vi "Calibration Process.vi"() -> ()   [LabVIEW 2016]
uses:
  <vilib>/vision/Calibration.llb/Correction Learn Setup.ctl
  <vilib>/vision/Calibration.llb/Distortion Model Types.ctl
  <vilib>/vision/Calibration.llb/Error Statistics.ctl
  <vilib>/vision/Calibration.llb/Distortion Model.ctl
  <vilib>/vision/NI_Vision_Development_Module.lvlib
panel:
  out "Error Statistics":T1 {"% Distortion" format="%#_2g"; "Standard Deviation" format="%#_2g"; "Mean Error" format="%#_2g"; "Maximum Error" format="%#_2g"}
  out "Error Map":sgl[][](array[numeric]) format="%.4f"
  out "Calibration Axis Info":T2={"Origin Pixel"={"X"=0.0, "Y"=0.0}, "Angle Relative to Horizontal (deg)"=0.0, "X Axis Pixel"={"X"=0.0, "Y"=0.0}, "Axis Reference"=1} {"X Axis Pixel"."Y" format="%.2f"; "X Axis Pixel"."X" format="%.2f"; "Axis Reference" items=["Direct", "Indirect"]; "Angle Relative to Horizontal (deg)" format="%.2f"; "Origin Pixel"."Y" format="%.2f"; "Origin Pixel"."X" format="%.2f"}
  out "Calibration Learn Setup":T3={"Method"=4, "Distortion"=-1, "Corrected Image Scaling"=0, "Corrected Image Learn ROI"=0, "Learn Correction Table?"=FALSE} {"Distortion" items=["None"=-1, "Polynomial"=0, "Division"=1]; "Corrected Image Learn ROI" items=["Full Image ", "Calibration ROI", "ROI", "Calibration AND ROI", "Calibration OR ROI"]; "Corrected Image Scaling" items=["Scale to Preserve Area", "Scale to Fit"]; "Method" items=["Perspective", "Microplane", "Simple", "Corrected", "None"]}
  out "Src":T5(plugin-control)
  out "Bin":T5(plugin-control)
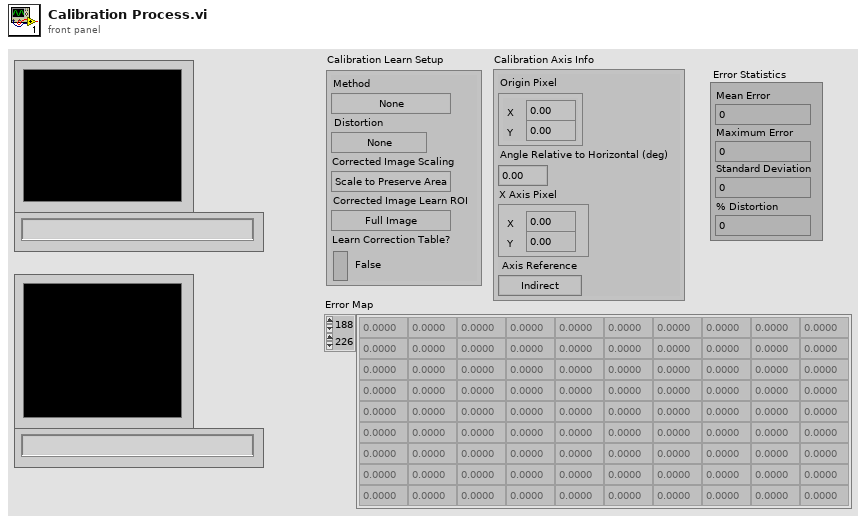
[diagram p1: front panel]
types:
  T1 = typedef "Error Statistics.ctl" = cluster{"Mean Error":dbl, "Maximum Error":dbl, "Standard Deviation":dbl, "% Distortion":dbl}
  T2 = cluster{"Origin Pixel":cluster{"X":sgl, "Y":sgl}, "Angle Relative to Horizontal (deg)":sgl, "X Axis Pixel":cluster{"X":sgl, "Y":sgl}, "Axis Reference":u32}
  T3 = typedef "Correction Learn Setup.ctl" = cluster{"Method":u32, "Distortion":T4, "Corrected Image Scaling":u32, "Corrected Image Learn ROI":u32, "Learn Correction Table?":bool}
  T4 = typedef "Distortion Model Types.ctl" = i32
  T5 = typedef "IMAQ Image.ctl" = refnum<image>
  T6 = typedef "Distortion Model.ctl" = cluster{"Distortion Model":T4, "Polynomial Model Setup":cluster{"Radial Coefficient":u32, "Tangential Coefficients ":bool}}
  T7 = typedef "Image Unit" = enum32{"Undefined", "Angström", "Micrometer", "Millimeter", "Centimeter", "Meter", "Kilometer", "Microinch", "Inch", "Feet", "Nautical miles", "Standard miles", "Steps"}
  T8 = typedef "Calibration Reference Points.ctl" = cluster{"Pixel Coordinates":cluster{"X":dbl, "Y":dbl}[], "Real World Coordinates":cluster{"X":dbl, "Y":dbl}[], "Unit":T7, "Image Size":cluster{"X":u32, "Y":u32}}
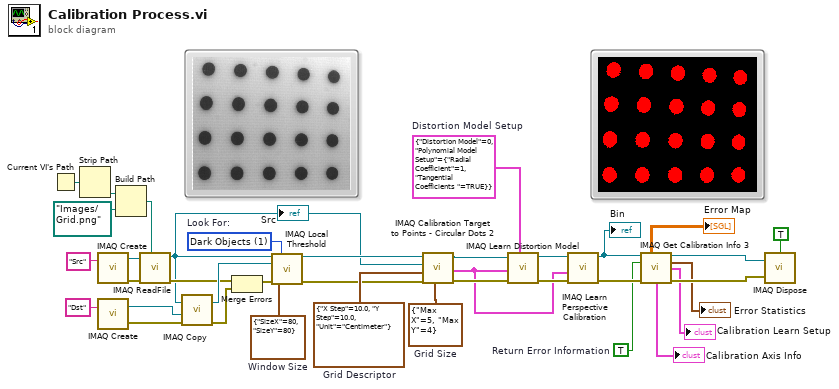
[diagram p0: block diagram]
diagram:
  w7 = TRUE  # Return Error Information
  w25 = T6 {"Distortion Model"=0, "Polynomial Model Setup"={"Radial Coefficient"=1, "Tangential Coefficients "=TRUE}}  # Distortion Model Setup
  w26 = cluster{"SizeX":i32, "SizeY":i32} {"SizeX"=80, "SizeY"=80}  # Window Size
  w27 = u32 1 items=["Bright Objects", "Dark Objects"]  # Look For:
  w28 = cluster{"Max X":u32, "Max Y":u32} {"Max X"=5, "Max Y"=4}  # Grid Size
  w30 = cluster{"X Step":sgl, "Y Step":sgl, "Unit":T7} {"X Step"=10.0, "Y Step"=10.0, "Unit"=enum."Centimeter"}  # Grid Descriptor
  n1 = Current VI's Path() -> (path=w33:path)
  n2 = Strip Path(path=w33) -> (stripped path=w32:path)  [unwired: 1 out]
  n3 = call "IMAQ Create"("Image Name"="Src") -> ("New Image"=w37:T5, "error out"=w36:errorcluster)  [unwired: 4 in]
  n4 = call "IMAQ Create"("Image Name"="Dst") -> ("New Image"=w15:T5, "error out"=w16:errorcluster)  [unwired: 4 in]
  n5 = Build Path(base path=w32, name or relative path=path "Images/Grid.png" ("prompt")) -> (appended path=w31:path)
  n6 = call "IMAQ ReadFile"("File Path"=w31, "error in (no error)"=w36, "Image"=w37) -> ("error out"=w12:errorcluster, "Image Out"=w6:T5)  [unwired: 4 in, 3 out]
  "Src" <- w6
  n7 = call "IMAQ Copy"("error in (no error)"=w16, "Image Dst"=w15, "Image Src"=w6) -> ("error out"=w11:errorcluster, "Image Dst Out"=w14:T5)  [unwired: 3 in]
  n8 = Merge Errors(w12, w11) -> (w10:errorcluster)
  n9 = call "IMAQ Local Threshold"("Image Src"=w6, "Look For (Bright Objects)"=w27, "Image Dst"=w14, "Window Size (32x32)"=w26, "error in (no error)"=w10) -> ("Image Dst Out"=w13:T5, "error out"=w22:errorcluster)  [unwired: 9 in]
  n10 = call "IMAQ Calibration Target to Points - Circular Dots 2"("Grid Size"=w28, "error in (no error)"=w22, "Grid Descriptor"=w30, "Grayscale Image"=w6, "Target Image"=w13) -> ("error out"=w21:errorcluster, "Reference Points"=w20:T8, "Target Image (dup)"=w5:T5)  [unwired: 4 in]
  n11 = call "IMAQ Learn Distortion Model"("Distortion Model Setup"=w25, "error in (no error)"=w21, "Reference Points"=w20, "Calibration Template Image"=w5) -> ("error out"=w24:errorcluster, "Calibration Template Image Out"=w9:T5)  [unwired: 2 in, 4 out]
  n12 = call "IMAQ Learn Perspective Calibration"("error in (no error)"=w24, "Reference Points"=w20, "Calibration Template Image"=w9) -> ("error out"=w23:errorcluster, "Calibration Template Image Out"=w8:T5)  [unwired: 1 in, 6 out]
  "Bin" <- w8
  n13 = call "IMAQ Get Calibration Info 3"("Calibration Template Image"=w8, "Return Error Information (False)"=w7, "error in (no error)"=w23) -> ("Error Map"=→"Error Map":sgl[][], "Calibration Template Image (duplicate)"=w18:T5, "Error Statistics"=→"Error Statistics":T1, "Calibration Learn Setup"=→"Calibration Learn Setup":T3, "Calibration Axis Info"=→"Calibration Axis Info":T2, "error out"=w19:errorcluster)  [unwired: 4 in, 3 out]
  n14 = call "IMAQ Dispose"("All Images? (No)"=TRUE, "Image"=w18, "error in (no error)"=w19) -> ()  [unwired: 3 in, 1 out]
